vi "SetCaptureFrames.vi"(8 "error in (no error)":errorcluster, 10 "Setting.FramesToCapture":i32, 11 "Camera_Prime95B in":refnum<class "Camera_Prime95B.lvclass">) -> (0 "error out":errorcluster, 3 "Camera_Prime95B out":refnum<class "Camera_Prime95B.lvclass">)   [LabVIEW 2020, in "Camera_Prime95B.lvlib" / "Camera_Prime95B.lvclass"]
uses:
  Camera_Prime95B.lvclass
  Camera_Prime95B.lvclass/Camera_Prime95B.ctl
  E:/Development/DevHardSoftware/MicroscopyFramework/Model/Hardware Layer/Real Hardware/Camera_Prime95B/Camera_Prime95B/Dependencies/PVCamNET.dll
  Dependencies/PVCamNET.dll
  Hardware Abstraction Layer/Component/Camera/Camera/Camera.lvclass
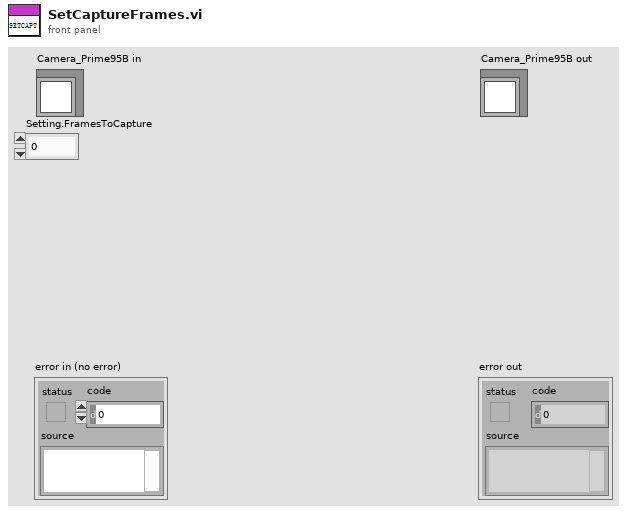
[diagram p1: front panel]
types:
  T1 = typedef "Device.lvlib/DeviceStatus.ctl" = i32
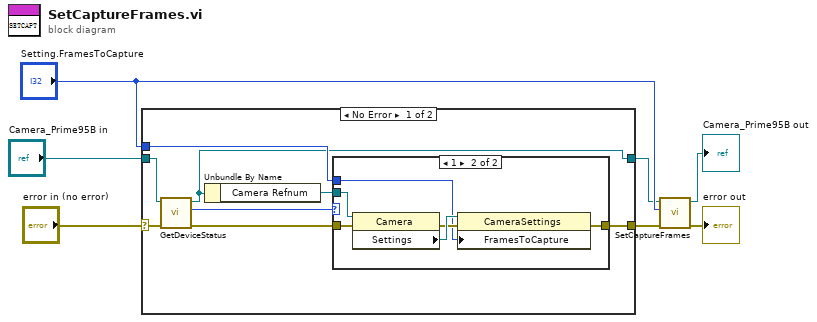
[diagram p0: block diagram]
diagram:
  n1 = case shown="No Error" "error in (no error)" {
    selector: "error in (no error)" -> [w13 w24]
    tunnel: [w14 w24] -> w3
    tunnel: "Camera_Prime95B in" -> [w12 w23]
    tunnel: "Setting.FramesToCapture" -> [w15 _]
    tunnel: [w8 w23] -> w1
    frame No Error {
      n2 = call-dynamic "GetDeviceStatus.vi"("error in (no error)"=w13, "Camera_Prime95B in"=w12) -> ("error out"=w10:errorcluster, "Status"=w11:T1, "Camera_Prime95B out"=w8:refnum<class "Camera_Prime95B.lvclass">)  [unwired: 7 in]
      n3 = Unbundle By Name(w8) -> ("Camera Refnum"=w9:refnum<k24>)
      n4 = case shown="1" w11 {
        tunnel: [w16 w22] -> w14
        tunnel: w9 -> [_ w19]
        tunnel: w15 -> [_ w18]
        tunnel: w10 -> [w16 w17]
        frame 0, Default {
        }
        frame 1 {
          n5 = property class="Camera"(reference=w19, error in=w17) -> (error out=w20:errorcluster, "Settings"=w21:refnum<k24>)  [unwired: 1 out]
          n6 = property class="CameraSettings"(reference=w21, error in=w20, "FramesToCapture"=w18) -> (error out=w22:errorcluster)  [unwired: 1 out]
        }
      }
    }
    frame Error {
    }
  }
  n7 = call-parent "SetCaptureFrames.vi"("error in (no error)"=w3, "Setting.FramesToCapture"="Setting.FramesToCapture", "Camera in"=w1) -> ("error out"=→"error out":errorcluster, "Camera out"=→"Camera_Prime95B out":refnum<class "Camera_Prime95B.lvclass">)  [unwired: 7 in]
